vi "Read Driver Joystick.vi"   [LabVIEW 2020]
uses:
  <vilib>/Rock Robotics/WPI/Utilities/WPI_GetSetVariantRefNum.vi
  <vilib>/Rock Robotics/Network Tables/NT Write Numeric Array.vi
  <vilib>/Rock Robotics/Network Tables/NT Write Boolean Array.vi
  Framework/Robot Global Data.vi
types:
  T1 = enum16{"0", "1", "2", "3", "4", "5", "6", "7", "8", "9", "10", "11"}
  T2 = typedef "WPI_JoystickDevRef.ctl" = cluster{"Device":T3}
  T3 = typedef "WPI_JoystickDeviceEnum.ctl" = enum16{"USB 0", "USB 1", "USB 2", "USB 3", "USB 4", "USB 5"}
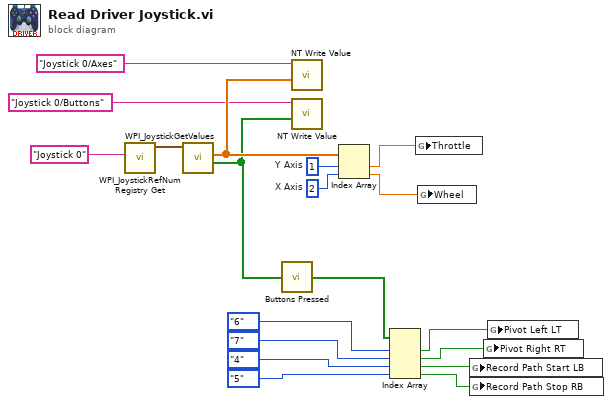
[diagram p0: block diagram]
diagram:
  w10 = 2  # X Axis
  w11 = 1  # Y Axis
  n1 = call <vilib>:"WPI_JoystickRefNum Registry Get.vi"("refnum name"="Joystick 0") -> ("JoystickDevRef"=w16:T2)  [unwired: 9 in, 1 out]
  n2 = call <vilib>:"WPI_JoystickGetValues.vi"("JoystickDevRef"=w16) -> ("Buttons"=w14:bool[], "Axes"=w19:dbl[])  [unwired: 6 in, 3 out]
  n3 = call "Buttons Pressed.vi"("Button Values"=w14) -> ("Button Presses"=w9:bool[])
  n4 = call-poly <vilib>:"NT Write Value.vi"("Numeric Array"=w19, "Name"="Joystick 0/Axes") -> ()  [unwired: 9 in, 1 out]
  n5 = call-poly <vilib>:"NT Write Value.vi"("Boolean Array"=w14, "Name"="Joystick 0/Buttons") -> ()  [unwired: 9 in, 1 out]
  n6 = Index Array(array=w19, index #1=w11, index #2=w10) -> (element #1=w13:dbl, element #2=w12:dbl)
  n7 = Index Array(array=w9, index #1=T1."6", index #2=T1."7", index #3=T1."4", index #4=T1."5") -> (element #1=w5:bool, element #2=w6:bool, element #3=w8:bool, element #4=w7:bool)
  n8 = global write "Robot Global Data.vi" "Throttle"(w13) -> ()
  n9 = global write "Robot Global Data.vi" "Wheel"(w12) -> ()
  n10 = global write "Robot Global Data.vi" "Record Path Start LB"(w8) -> ()
  n11 = global write "Robot Global Data.vi" "Record Path Stop RB"(w7) -> ()
  n12 = global write "Robot Global Data.vi" "Pivot Right RT"(w6) -> ()
  n13 = global write "Robot Global Data.vi" "Pivot Left LT"(w5) -> ()
